vi "Main.vi"(10 "COMport name":refnum<visa-resource-name>, 11 "Module Admin":refnum<class "Delacor_lib_QMH_Module Admin.lvclass">) -> ()   [LabVIEW 2018, in "MB 01 switches Module.lvlib"]
doc: "This template is based off of the Queued Message Handler design pattern and the Queued Message Handler project template that ships with LabVIEW.\n\nThe main difference is that the queue is private to this module and communication between modules is performed via Broadcast and Request events.\n\nRequest events are wrapped in public API methods and are handled in the Event Handling Loop (EHL) of this VI. Any module can register for Broadcast events sent by this module. The EHL generates messages based on user interface actions.\n\nThe Message Handling Loop (MHL) processes messages generated by the EHL, or by other messages. The messages are string values, so new messages can be added easily to the Message Cases case structure in the MHL. Each message cluster can also provide an optional value for Message Data, which is a variant that can be converted to whatever message-specific data is required.\n_____\nBased on DQMH Project Template 6.0.0.91."
uses:
  MB 01 switches Module.lvlib
  <vilib>/Delacor/Delacor QMH/Libraries/Module Admin_class/Delacor_lib_QMH_Module Admin.lvclass
  Module Data--cluster.ctl
  <vilib>/NI/Modbus Library/API/Master/Modbus Master.lvclass
  <vilib>/Delacor/Delacor QMH/Libraries/Message Queue_class/Delacor_lib_QMH_Message Queue.lvclass/Delacor_lib_QMH_Message Queue.ctl
  Stop Argument--cluster.ctl
  <vilib>/Delacor/Delacor QMH/Libraries/Module Admin_class/Delacor_lib_QMH_Module Admin.lvclass/Delacor_lib_QMH_Module Admin.ctl
  MB01 Open Argument--cluster.ctl
  demux1-10_chan0 Argument--cluster.ctl
  MB01_eMICs Argument--cluster.ctl
  MB01 Close Argument--cluster.ctl
  JIG Reset Argument--cluster.ctl
  Read JIG trigger Argument--cluster.ctl
  Read JIG trigger (Reply Payload)--cluster.ctl
  SC enable OFF Argument--cluster.ctl
  demux1-10_chan1 Argument--cluster.ctl
  demux1-10_chan2 Argument--cluster.ctl
  demux1-10_chan3 Argument--cluster.ctl
  demux1-10_chan4 Argument--cluster.ctl
  demux1-10_chan5 Argument--cluster.ctl
  demux1-10_chan6 Argument--cluster.ctl
  demux1-10_chan7 Argument--cluster.ctl
  demux1-10_chan8 Argument--cluster.ctl
  demux1-10_chan9 Argument--cluster.ctl
  demux1-10_chan10 Argument--cluster.ctl
  SC enable ON Argument--cluster.ctl
  SET trigger value Argument--cluster.ctl
  <vilib>/Utility/miscctls.llb/LVPointTypeDef.ctl
  Instrument Drivers/LV_driver_MBrelay/type defs/FGV enum.ctl
  <vilib>/Delacor/Delacor QMH/Libraries/Message Queue_class/Delacor_lib_QMH_Enqueue Message (Single).vi
  <vilib>/Delacor/Delacor QMH/Libraries/Module Admin_class/Delacor_lib_QMH_Get External Launch.vi
  <vilib>/Utility/error.llb/Error Cluster From Error Code.vi
  <vilib>/ErrorRing/Error Ring.xnode
  <vilib>/Delacor/Delacor QMH/Libraries/Message Queue_class/Delacor_lib_QMH_Message Queue.lvclass
  Instrument Drivers/LV_driver_MBrelay/MB Relay.lvlib
panel:
  out "trigger value":bool
  out "error out":errorcluster
  out "Status":string
  in  "Simulate MHL Error":bool
  in  "Simulate EHL Error":bool
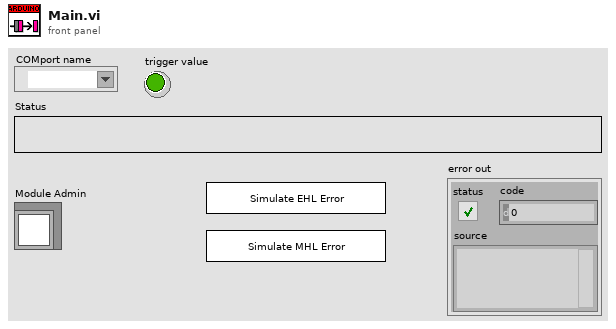
[diagram p1: front panel]
types:
  T1 = typedef "MB 01 switches Module.lvlib/Request Events--cluster.ctl" = cluster{"Stop Module":refnum<user-event>, "Show Panel":refnum<user-event>, "Hide Panel":refnum<user-event>, "Get Module Execution Status":refnum<user-event>, "Show Diagram":refnum<user-event>, "MB01 Open":refnum<user-event>, "demux1-10_chan0":refnum<user-event>, "MB01_eMICs":refnum<user-event>, "MB01 Close":refnum<user-event>, "JIG Reset":refnum<user-event>, "Read JIG trigger":refnum<user-event>, "SC enable OFF":refnum<user-event>, "demux1-10_chan1":refnum<user-event>, "demux1-10_chan2":refnum<user-event>, "demux1-10_chan3":refnum<user-event>, "demux1-10_chan4":refnum<user-event>, "demux1-10_chan5":refnum<user-event>, "demux1-10_chan6":refnum<user-event>, "demux1-10_chan7":refnum<user-event>, "demux1-10_chan8":refnum<user-event>, "demux1-10_chan9":refnum<user-event>, "demux1-10_chan10":refnum<user-event>, "SC enable ON":refnum<user-event>, "SET trigger value":refnum<user-event>}
  T2 = typedef "MB 01 switches Module.lvlib/Module Data--cluster.ctl" = cluster{"Status":string, "VISA resource name":refnum<visa-resource-name>, "Modbus Master out":refnum<class "Modbus Master.lvclass">}
  T3 = enum32{"invalid lock state", "Not Locked", "Locked (No Password)", "Password-protected"}
  T4 = typedef "MB 01 switches Module.lvlib/Stop Argument--cluster.ctl" = cluster{"Origin":string, "Exit via Stop Module Req?":bool, "Wait for Module to stop?":bool}
  T5 = typedef "MB 01 switches Module.lvlib/MB01 Open Argument--cluster.ctl" = cluster{"VISA resource name":refnum<visa-resource-name>}
  T6 = typedef "MB 01 switches Module.lvlib/demux1-10_chan0 Argument--cluster.ctl" = cluster{"demux1_10(x6)_encode":enum16{"demux1_10_channel0", "demux1_10_channel1", "demux1_10_channel2", "demux1_10_channel3", "demux1_10_channel4", "demux1_10_channel5", "demux1_10_channel6", "demux1_10_channel7", "demux1_10_channel8", "demux1_10_channel9", "demux1_10_channel10"}}
  T7 = typedef "MB 01 switches Module.lvlib/MB01_eMICs Argument--cluster.ctl" = cluster{"Array":bool[]}
  T8 = typedef "MB 01 switches Module.lvlib/MB01 Close Argument--cluster.ctl" = cluster{"Boolean":bool}
  T9 = typedef "MB 01 switches Module.lvlib/JIG Reset Argument--cluster.ctl" = cluster{"Boolean":bool}
  T10 = typedef "MB 01 switches Module.lvlib/Read JIG trigger Argument--cluster.ctl" = cluster{"Wait Notifier":refnum<notifier>, "wait for reply":bool}
  T11 = typedef "MB 01 switches Module.lvlib/SC enable OFF Argument--cluster.ctl" = cluster{"Boolean":bool}
  T12 = typedef "MB 01 switches Module.lvlib/demux1-10_chan1 Argument--cluster.ctl" = cluster{"Boolean":bool}
  T13 = typedef "MB 01 switches Module.lvlib/demux1-10_chan2 Argument--cluster.ctl" = cluster{"Boolean":bool}
  T14 = typedef "MB 01 switches Module.lvlib/demux1-10_chan3 Argument--cluster.ctl" = cluster{"Boolean":bool}
  T15 = typedef "MB 01 switches Module.lvlib/demux1-10_chan4 Argument--cluster.ctl" = cluster{"Boolean":bool}
  T16 = typedef "MB 01 switches Module.lvlib/demux1-10_chan5 Argument--cluster.ctl" = cluster{"Boolean":bool}
  T17 = typedef "MB 01 switches Module.lvlib/demux1-10_chan6 Argument--cluster.ctl" = cluster{"Boolean":bool}
  T18 = typedef "MB 01 switches Module.lvlib/demux1-10_chan7 Argument--cluster.ctl" = cluster{"Boolean":bool}
  T19 = typedef "MB 01 switches Module.lvlib/demux1-10_chan8 Argument--cluster.ctl" = cluster{"Boolean":bool}
  T20 = typedef "MB 01 switches Module.lvlib/demux1-10_chan9 Argument--cluster.ctl" = cluster{"Boolean":bool}
  T21 = typedef "MB 01 switches Module.lvlib/demux1-10_chan10 Argument--cluster.ctl" = cluster{"Boolean":bool}
  T22 = typedef "MB 01 switches Module.lvlib/SC enable ON Argument--cluster.ctl" = cluster{"Boolean":bool}
  T23 = typedef "MB 01 switches Module.lvlib/SET trigger value Argument--cluster.ctl" = cluster{"Boolean":bool}
  T24 = typedef "LVPointTypeDef.ctl" = cluster{"Horizontal":i16, "Vertical":i16}
  T25 = enum32{"Invalid", "Standard", "Closed", "Hidden", "Minimized", "Maximized"}
  T26 = typedef "MB Relay.lvlib/FGV enum.ctl" = enum16{"Write", "Init FGV", "Read", "All OFF", "All ON"}
  T27 = enum16{"demux1_10_channel0", "demux1_10_channel1", "demux1_10_channel2", "demux1_10_channel3", "demux1_10_channel4", "demux1_10_channel5", "demux1_10_channel6", "demux1_10_channel7", "demux1_10_channel8", "demux1_10_channel9", "demux1_10_channel10"}
  T28 = typedef "MB 01 switches Module.lvlib/Read JIG trigger (Reply Payload)--cluster.ctl" = cluster{"Trigger?":bool, "Read JIG trigger_error":errorcluster}
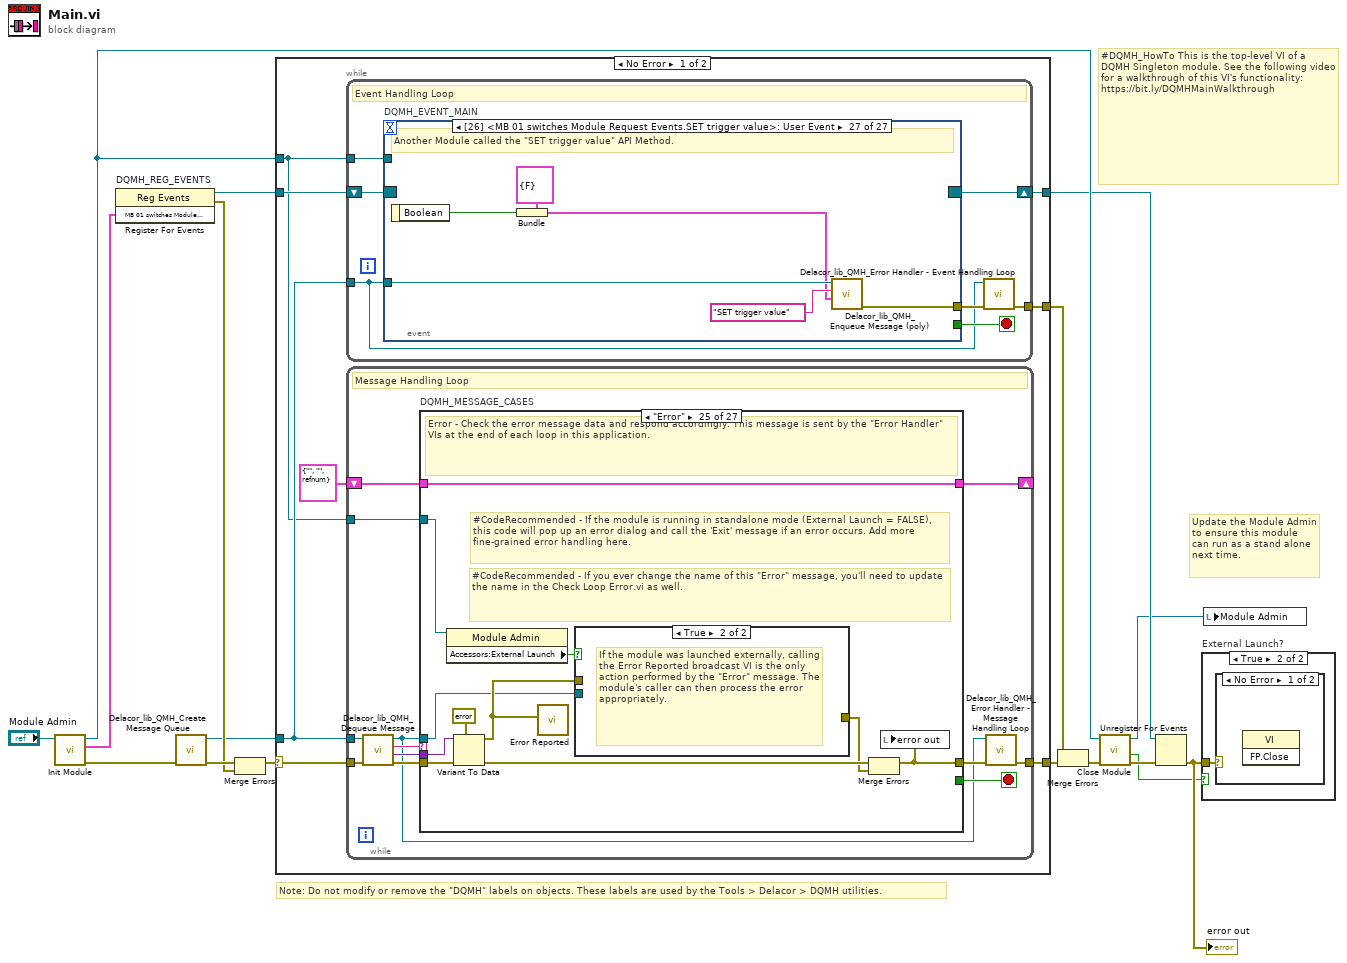
[diagram p0: block diagram]
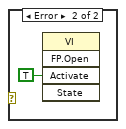
[diagram p3: hidden frame]
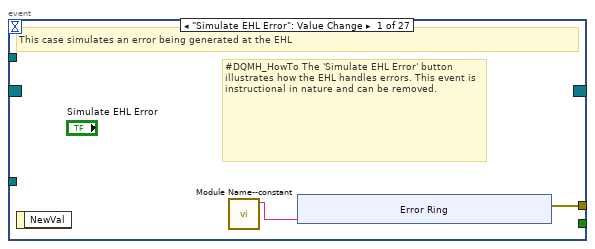
[diagram p4: hidden frame]
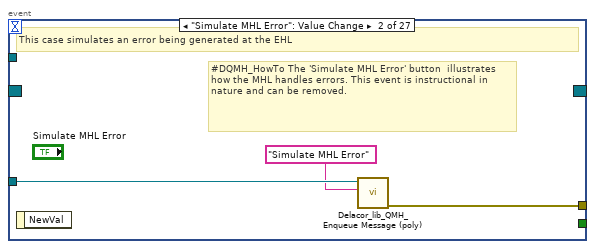
[diagram p5: hidden frame]
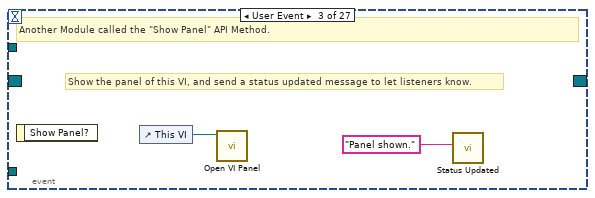
[diagram p6: hidden frame]
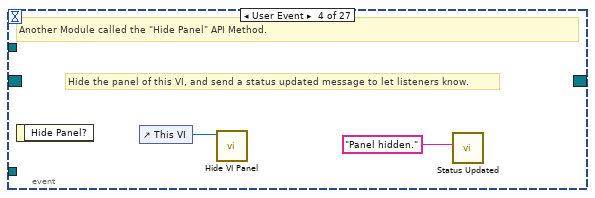
[diagram p7: hidden frame]
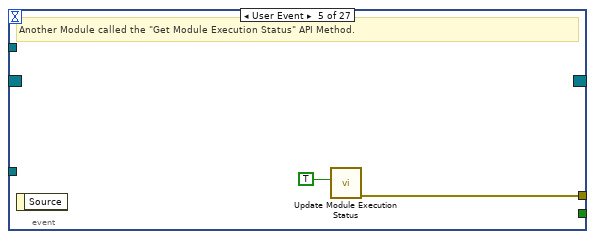
[diagram p8: hidden frame]
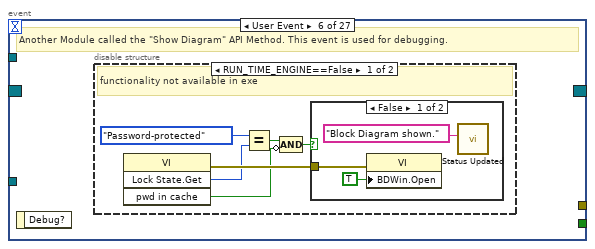
[diagram p9: hidden frame]
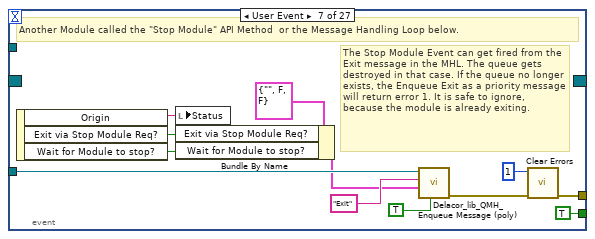
[diagram p12: hidden frame]
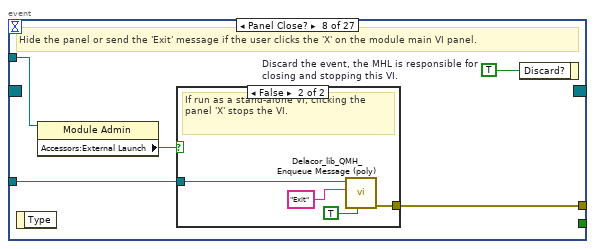
[diagram p13: hidden frame]
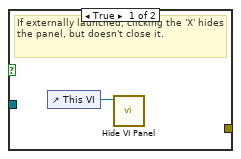
[diagram p14: hidden frame]
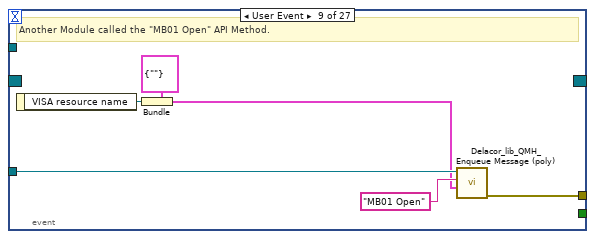
[diagram p15: hidden frame]
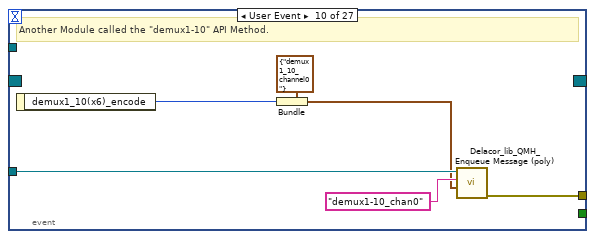
[diagram p16: hidden frame]
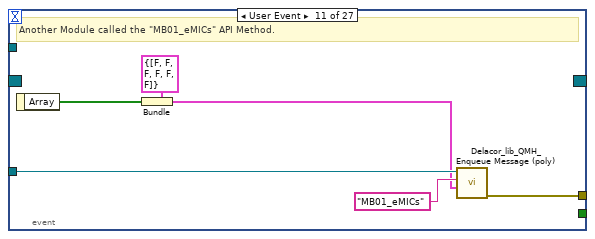
[diagram p17: hidden frame]
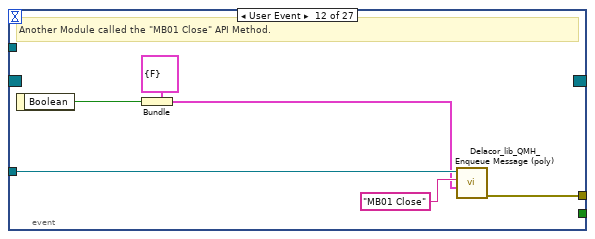
[diagram p18: hidden frame]
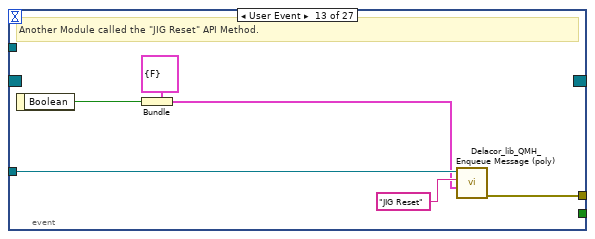
[diagram p19: hidden frame]
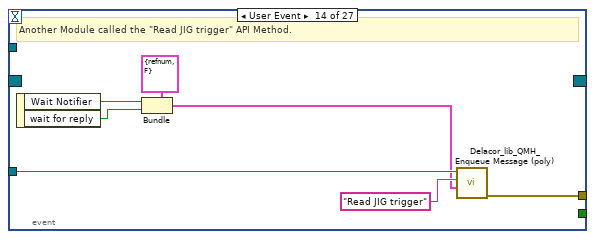
[diagram p20: hidden frame]
diagram:
  # "#DQMH_HowTo This is the top-level VI of a DQMH Singleton module. See the following video for a walkthrough of this VI's functionality: https://bit.ly/DQMHMainWalkthrough"
  # "Note: Do not modify or remove the \"DQMH\" labels on objects. These labels are used by the Tools > Delacor > DQMH utilities."
  # "Update the Module Admin to ensure this module can run as a stand alone next time."
  n1 = call "Init Module.vi"("Singleton Module Admin in"="Module Admin") -> ("error out"=w16:errorcluster, "MB 01 switches Module Request Events"=w5:T1, "Singleton Module Admin out"=w8:refnum<class "Delacor_lib_QMH_Module Admin.lvclass">)  [unwired: 8 in]
  n2 = register-events "DQMH_REG_EVENTS"(w5) -> (reference out=w6:refnum<event-registration>, error out=w9:errorcluster)  [unwired: 2 in]
  n3 = call <vilib>:"Delacor_lib_QMH_Create Message Queue.vi"("error in"=w16) -> ("error out"=w11:errorcluster, "Message Queue"=w4:refnum<class "Delacor_lib_QMH_Message Queue.lvclass">)  [unwired: 9 in]
  n4 = Merge Errors(w11, w9) -> (w10:errorcluster)
  n5 = case shown="No Error" w10 {
    selector: w10 -> [w23 w534]
    tunnel: [w25 w533] -> w17
    tunnel: [w22 w539] -> w7
    tunnel: w6 -> [w20 w539]
    tunnel: w4 -> [w19 w532]
    tunnel: [w24 _] -> w14
    tunnel: w8 -> [w18 w535]
    frame No Error {
      n6 = while {
        tunnel: w19 -> [w26]
        shift-right: [w29] -> w22
        shift-left: w20 -> [w30]
        tunnel: [w31] -> w24
        tunnel: w18 -> [w27]
        stop <- w28 stop-if-true
        # "Event Handling Loop"
        n7 = event "DQMH_EVENT_MAIN" shown="[26] <MB 01 switches Module Request Events.SET trigger value>: User Event" {
          selector: w30 -> [_ _ _ _ _ _ _ _ _ _ _ _ _ _ _ _ _ _ _ _ _ _ _ _ _ _ _]
          dyn-events: [_ _ _ _ _ _ _ _ _ _ _ _ _ _ _ _ _ _ _ _ _ _ _ _ _ _ _] -> w29
          timeout: _ -> [_ _ _ _ _ _ _ _ _ _ _ _ _ _ _ _ _ _ _ _ _ _ _ _ _ _ _]
          tunnel: [_ _ _ _ _ _ TRUE ("Discard?") _ _ _ _ _ _ _ _ _ _ _ _ _ _ _ _ _ _ _ _] -> w28
          tunnel: w26 -> [_ w43 _ _ _ _ w67 w74 w87 w93 w99 w105 w111 w118 w124 w130 w136 w142 w148 w154 w160 w166 w172 w178 w184 w190 w196]
          tunnel: [w34 w44 _ _ w50 _ w70 w76 w82 w88 w94 w100 w106 w112 w119 w125 w131 w137 w143 w149 w155 w161 w167 w173 w179 w185 w191] -> w32
          tunnel: w27 -> [_ _ _ _ _ _ _ w73 _ _ _ _ _ _ _ _ _ _ _ _ _ _ _ _ _ _ _]
          event "Simulate EHL Error": Value Change {
            # "#DQMH_HowTo The 'Simulate EHL Error' button  illustrates how the EHL handles errors. This event is instructional in nature and can be removed."
            # "This case simulates an error being generated at the EHL"
            n8 = event-data() -> ()  [unwired: 1 in, 1 out]
            n9 = call "Module Name--constant.vi"() -> ("Module Name"=w33:string)  [unwired: 11 in]
            n10 = xnode "Error Ring"("parameter 0"=w33) -> ("error out"=w34:errorcluster)
          }
          event "Simulate MHL Error": Value Change {
            # "#DQMH_HowTo The 'Simulate MHL Error' button  illustrates how the MHL handles errors. This event is instructional in nature and can be removed."
            # "This case simulates an error being generated at the EHL"
            n11 = event-data() -> ()  [unwired: 1 in, 1 out]
            n12 = call-poly <vilib>:"Delacor_lib_QMH_Enqueue Message (poly).vi"("Message"="Simulate MHL Error", "Message Queue in"=w43) -> ("error out"=w44:errorcluster)  [unwired: 8 in, 1 out]
          }
          event User Event {
            # "Show the panel of this VI, and send a status updated message to let listeners know."
            # "Another Module called the \"Show Panel\" API Method."
            n13 = event-data() -> ()  [unwired: 1 in, 1 out]
            n14 = control-ref of="This VI"() -> (w46:refnum<vi>)
            n15 = call "Open VI Panel.vi"("VI"=w46) -> ()  [unwired: 10 in, 1 out]
            n16 = call "Status Updated.vi"("Status"="Panel shown." ("format string")) -> ()  [unwired: 10 in, 1 out]
          }
          event User Event {
            # "Hide the panel of this VI, and send a status updated message to let listeners know."
            # "Another Module called the \"Hide Panel\" API Method."
            n17 = event-data() -> ()  [unwired: 1 in, 1 out]
            n18 = control-ref of="This VI"() -> (w48:refnum<vi>)
            n19 = call "Hide VI Panel.vi"("VI"=w48) -> ()  [unwired: 10 in, 1 out]
            n20 = call "Status Updated.vi"("Status"="Panel hidden." ("format string")) -> ()  [unwired: 10 in, 1 out]
          }
          event User Event {
            # "Another Module called the \"Get Module Execution Status\" API Method."
            n21 = event-data() -> ()  [unwired: 1 in, 1 out]
            n22 = call "Update Module Execution Status.vi"("Running?"=TRUE) -> ("error out"=w50:errorcluster)  [unwired: 10 in]
          }
          event User Event {
            # "Another Module called the \"Show Diagram\" API Method. This event is used for debugging."
            n23 = event-data() -> ()  [unwired: 1 in, 1 out]
            n24 = disable-structure shown="RUN_TIME_ENGINE==False" {
              frame condition #0 (active) {
                # "functionality not available in exe"
                n25 = invoke class="VI" method="Lock State.Get"() -> (error out=w56:errorcluster, "Get Lock State"=w55:T3, "pwd in cache"=w52:bool)  [unwired: 4 in, 1 out]
                n26 = Equal?(x=T3."Password-protected", y=w55) -> (x = y?=w53:bool)
                n27 = Compound Arithmetic op=AND(w53, invert w52) -> (w51:bool)
                n28 = case shown="False" w51 {
                  tunnel: w56 -> [w59 _]
                  frame False {
                    n29 = property class="VI"(error in=w59, "BDWin.Open"=TRUE ("Block Diagram Window:Open")) -> ()  [unwired: 1 in, 2 out]
                    n30 = call "Status Updated.vi"("Status"="Block Diagram shown." ("format string")) -> ()  [unwired: 10 in, 1 out]
                  }
                  frame True {
                    # "Password-protected VI, and the password is not in the cache. Do not show the diagram."
                  }
                }
              }
              frame condition #1 {
              }
            }
          }
          event User Event {
            # "The Stop Module Event can get fired from the Exit message in the MHL. The queue gets destroyed in that case. If the queue no longer exists, the Enqueue Exit as a priority message will return error 1. It is safe to ignore, because the module is already exiting."
            # "Another Module called the \"Stop Module\" API Method  or the Message Handling Loop below."
            n31 = event-data() -> ("Origin"=w66:string, "Exit via Stop Module Req?"=w62:bool, "Wait for Module to stop?"=w61:bool)  [unwired: 1 in]
            n32 = local write "Status"(w66) -> ()
            n33 = Bundle By Name(cluster=T4 {"Origin"="", "Exit via Stop Module Req?"=FALSE, "Wait for Module to stop?"=FALSE} ("Stop Argument"), "Exit via Stop Module Req?"=w62, "Wait for Module to stop?"=w61) -> (w60:T4)
            n34 = call-poly <vilib>:"Delacor_lib_QMH_Enqueue Message (poly).vi"("Priority Message? (F)"=TRUE, "Message Data"=w60, "Message"="Exit", "Message Queue in"=w67) -> ("error out"=w71:errorcluster)  [unwired: 6 in, 1 out]
            n35 = call <vilib>:"Clear Errors.vi"("error in (no error)"=w71, "specific error code to clear (0: all)"=1) -> ("error out"=w70:errorcluster)  [unwired: 4 in, 1 out]
          }
          event Panel Close? {
            w75 = TRUE  # Discard the event, the MHL is responsible for closing and stopping this VI.
            # "Hide the panel or send the 'Exit' message if the user clicks the 'X' on the module main VI panel."
            n36 = event-data() -> ()  [unwired: 1 in, 1 out]
            n37 = property class="Module Admin"(reference=w73) -> ("Accessors:External Launch"=w72:bool)  [unwired: 1 in, 2 out]
            n38 = case shown="False" w72 {
              tunnel: w74 -> [_ w80]
              tunnel: [_ w81] -> w76
              frame True {
                # "If externally launched, clicking the 'X' hides the panel, but doesn't close it."
                n39 = control-ref of="This VI"() -> (w77:refnum<vi>)
                n40 = call "Hide VI Panel.vi"("VI"=w77) -> ()  [unwired: 10 in, 1 out]
              }
              frame False {
                # "If run as a stand-alone VI, clicking the panel 'X' stops the VI."
                n41 = call-poly <vilib>:"Delacor_lib_QMH_Enqueue Message (poly).vi"("Priority Message? (F)"=TRUE, "Message"="Exit", "Message Queue in"=w80) -> ("error out"=w81:errorcluster)  [unwired: 7 in, 1 out]
              }
            }
            n42 = event-data("Discard?"=w75) -> ()  [unwired: 1 in, 1 out]
          }
          event User Event {
            # "Another Module called the \"MB01 Open\" API Method."
            n43 = event-data() -> ("VISA resource name"=w83:refnum<visa-resource-name>)  [unwired: 1 in]
            n44 = Bundle(cluster=T5 {"VISA resource name"=""} ("MB01 Open Argument"), "VISA resource name"=w83) -> (w84:T5)
            n45 = call-poly <vilib>:"Delacor_lib_QMH_Enqueue Message (poly).vi"("Message Data"=w84, "Message"="MB01 Open", "Message Queue in"=w87) -> ("error out"=w82:errorcluster)  [unwired: 7 in, 1 out]
          }
          event User Event {
            # "Another Module called the \"demux1-10\" API Method."
            n46 = event-data() -> ("demux1_10(x6)_encode"=w89:T27)  [unwired: 1 in]
            n47 = Bundle(cluster=T6 {"demux1_10(x6)_encode"=enum."demux1_10_channel0"} ("demux1-10 Argument"), "demux1_10(x6)_encode"=w89) -> (w90:T6)
            n48 = call-poly <vilib>:"Delacor_lib_QMH_Enqueue Message (poly).vi"("Message Data"=w90, "Message"="demux1-10_chan0", "Message Queue in"=w93) -> ("error out"=w88:errorcluster)  [unwired: 7 in, 1 out]
          }
          event User Event {
            # "Another Module called the \"MB01_eMICs\" API Method."
            n49 = event-data() -> ("Array"=w95:bool[])  [unwired: 1 in]
            n50 = Bundle(cluster=T7 {"Array"=[FALSE, FALSE, FALSE, FALSE, FALSE, FALSE]} ("MB01_eMICs Argument"), "Array"=w95) -> (w96:T7)
            n51 = call-poly <vilib>:"Delacor_lib_QMH_Enqueue Message (poly).vi"("Message Data"=w96, "Message"="MB01_eMICs", "Message Queue in"=w99) -> ("error out"=w94:errorcluster)  [unwired: 7 in, 1 out]
          }
          event User Event {
            # "Another Module called the \"MB01 Close\" API Method."
            n52 = event-data() -> ("Boolean"=w101:bool)  [unwired: 1 in]
            n53 = Bundle(cluster=T8 {"Boolean"=FALSE} ("MB01 Close Argument"), "Boolean"=w101) -> (w102:T8)
            n54 = call-poly <vilib>:"Delacor_lib_QMH_Enqueue Message (poly).vi"("Message Data"=w102, "Message"="MB01 Close", "Message Queue in"=w105) -> ("error out"=w100:errorcluster)  [unwired: 7 in, 1 out]
          }
          event User Event {
            # "Another Module called the \"JIG Reset\" API Method."
            n55 = event-data() -> ("Boolean"=w107:bool)  [unwired: 1 in]
            n56 = Bundle(cluster=T9 {"Boolean"=FALSE} ("JIG Reset Argument"), "Boolean"=w107) -> (w108:T9)
            n57 = call-poly <vilib>:"Delacor_lib_QMH_Enqueue Message (poly).vi"("Message Data"=w108, "Message"="JIG Reset", "Message Queue in"=w111) -> ("error out"=w106:errorcluster)  [unwired: 7 in, 1 out]
          }
          event User Event {
            # "Another Module called the \"Read JIG trigger\" API Method."
            n58 = event-data() -> ("Wait Notifier"=w114:refnum<notifier>, "wait for reply"=w113:bool)  [unwired: 1 in]
            n59 = Bundle(cluster=T10 {"Wait Notifier"=refnum, "wait for reply"=FALSE} ("Read JIG trigger Argument"), "Wait Notifier"=w114, "wait for reply"=w113) -> (w115:T10)
            n60 = call-poly <vilib>:"Delacor_lib_QMH_Enqueue Message (poly).vi"("Message Data"=w115, "Message"="Read JIG trigger", "Message Queue in"=w118) -> ("error out"=w112:errorcluster)  [unwired: 7 in, 1 out]
          }
          event User Event {
            # "Another Module called the \"SC enable OFF\" API Method."
            n61 = event-data() -> ("Boolean"=w120:bool)  [unwired: 1 in]
            n62 = Bundle(cluster=T11 {"Boolean"=FALSE} ("SC enable OFF Argument"), "Boolean"=w120) -> (w121:T11)
            n63 = call-poly <vilib>:"Delacor_lib_QMH_Enqueue Message (poly).vi"("Message Data"=w121, "Message"="SC enable OFF", "Message Queue in"=w124) -> ("error out"=w119:errorcluster)  [unwired: 7 in, 1 out]
          }
          event User Event {
            # "Another Module called the \"demux1-10_chan1\" API Method."
            n64 = event-data() -> ("Boolean"=w126:bool)  [unwired: 1 in]
            n65 = Bundle(cluster=T12 {"Boolean"=FALSE} ("demux1-10_chan1 Argument"), "Boolean"=w126) -> (w127:T12)
            n66 = call-poly <vilib>:"Delacor_lib_QMH_Enqueue Message (poly).vi"("Message Data"=w127, "Message"="demux1-10_chan1", "Message Queue in"=w130) -> ("error out"=w125:errorcluster)  [unwired: 7 in, 1 out]
          }
          event User Event {
            # "Another Module called the \"demux1-10_chan2\" API Method."
            n67 = event-data() -> ("Boolean"=w132:bool)  [unwired: 1 in]
            n68 = Bundle(cluster=T13 {"Boolean"=FALSE} ("demux1-10_chan2 Argument"), "Boolean"=w132) -> (w133:T13)
            n69 = call-poly <vilib>:"Delacor_lib_QMH_Enqueue Message (poly).vi"("Message Data"=w133, "Message"="demux1-10_chan2", "Message Queue in"=w136) -> ("error out"=w131:errorcluster)  [unwired: 7 in, 1 out]
          }
          event User Event {
            # "Another Module called the \"demux1-10_chan3\" API Method."
            n70 = event-data() -> ("Boolean"=w138:bool)  [unwired: 1 in]
            n71 = Bundle(cluster=T14 {"Boolean"=FALSE} ("demux1-10_chan3 Argument"), "Boolean"=w138) -> (w139:T14)
            n72 = call-poly <vilib>:"Delacor_lib_QMH_Enqueue Message (poly).vi"("Message Data"=w139, "Message"="demux1-10_chan3", "Message Queue in"=w142) -> ("error out"=w137:errorcluster)  [unwired: 7 in, 1 out]
          }
          event User Event {
            # "Another Module called the \"demux1-10_chan4\" API Method."
            n73 = event-data() -> ("Boolean"=w144:bool)  [unwired: 1 in]
            n74 = Bundle(cluster=T15 {"Boolean"=FALSE} ("demux1-10_chan4 Argument"), "Boolean"=w144) -> (w145:T15)
            n75 = call-poly <vilib>:"Delacor_lib_QMH_Enqueue Message (poly).vi"("Message Data"=w145, "Message"="demux1-10_chan4", "Message Queue in"=w148) -> ("error out"=w143:errorcluster)  [unwired: 7 in, 1 out]
          }
          event User Event {
            # "Another Module called the \"demux1-10_chan5\" API Method."
            n76 = event-data() -> ("Boolean"=w150:bool)  [unwired: 1 in]
            n77 = Bundle(cluster=T16 {"Boolean"=FALSE} ("demux1-10_chan5 Argument"), "Boolean"=w150) -> (w151:T16)
            n78 = call-poly <vilib>:"Delacor_lib_QMH_Enqueue Message (poly).vi"("Message Data"=w151, "Message"="demux1-10_chan5", "Message Queue in"=w154) -> ("error out"=w149:errorcluster)  [unwired: 7 in, 1 out]
          }
          event User Event {
            # "Another Module called the \"demux1-10_chan6\" API Method."
            n79 = event-data() -> ("Boolean"=w156:bool)  [unwired: 1 in]
            n80 = Bundle(cluster=T17 {"Boolean"=FALSE} ("demux1-10_chan6 Argument"), "Boolean"=w156) -> (w157:T17)
            n81 = call-poly <vilib>:"Delacor_lib_QMH_Enqueue Message (poly).vi"("Message Data"=w157, "Message"="demux1-10_chan6", "Message Queue in"=w160) -> ("error out"=w155:errorcluster)  [unwired: 7 in, 1 out]
          }
          event User Event {
            # "Another Module called the \"demux1-10_chan7\" API Method."
            n82 = event-data() -> ("Boolean"=w162:bool)  [unwired: 1 in]
            n83 = Bundle(cluster=T18 {"Boolean"=FALSE} ("demux1-10_chan7 Argument"), "Boolean"=w162) -> (w163:T18)
            n84 = call-poly <vilib>:"Delacor_lib_QMH_Enqueue Message (poly).vi"("Message Data"=w163, "Message"="demux1-10_chan7", "Message Queue in"=w166) -> ("error out"=w161:errorcluster)  [unwired: 7 in, 1 out]
          }
          event User Event {
            # "Another Module called the \"demux1-10_chan8\" API Method."
            n85 = event-data() -> ("Boolean"=w168:bool)  [unwired: 1 in]
            n86 = Bundle(cluster=T19 {"Boolean"=FALSE} ("demux1-10_chan8 Argument"), "Boolean"=w168) -> (w169:T19)
            n87 = call-poly <vilib>:"Delacor_lib_QMH_Enqueue Message (poly).vi"("Message Data"=w169, "Message"="demux1-10_chan8", "Message Queue in"=w172) -> ("error out"=w167:errorcluster)  [unwired: 7 in, 1 out]
          }
          event User Event {
            # "Another Module called the \"demux1-10_chan9\" API Method."
            n88 = event-data() -> ("Boolean"=w174:bool)  [unwired: 1 in]
            n89 = Bundle(cluster=T20 {"Boolean"=FALSE} ("demux1-10_chan9 Argument"), "Boolean"=w174) -> (w175:T20)
            n90 = call-poly <vilib>:"Delacor_lib_QMH_Enqueue Message (poly).vi"("Message Data"=w175, "Message"="demux1-10_chan9", "Message Queue in"=w178) -> ("error out"=w173:errorcluster)  [unwired: 7 in, 1 out]
          }
          event User Event {
            # "Another Module called the \"demux1-10_chan10\" API Method."
            n91 = event-data() -> ("Boolean"=w180:bool)  [unwired: 1 in]
            n92 = Bundle(cluster=T21 {"Boolean"=FALSE} ("demux1-10_chan10 Argument"), "Boolean"=w180) -> (w181:T21)
            n93 = call-poly <vilib>:"Delacor_lib_QMH_Enqueue Message (poly).vi"("Message Data"=w181, "Message"="demux1-10_chan10", "Message Queue in"=w184) -> ("error out"=w179:errorcluster)  [unwired: 7 in, 1 out]
          }
          event User Event {
            # "Another Module called the \"SC enable ON\" API Method."
            n94 = event-data() -> ("Boolean"=w186:bool)  [unwired: 1 in]
            n95 = Bundle(cluster=T22 {"Boolean"=FALSE} ("SC enable ON Argument"), "Boolean"=w186) -> (w187:T22)
            n96 = call-poly <vilib>:"Delacor_lib_QMH_Enqueue Message (poly).vi"("Message Data"=w187, "Message"="SC enable ON", "Message Queue in"=w190) -> ("error out"=w185:errorcluster)  [unwired: 7 in, 1 out]
          }
          event User Event {
            # "Another Module called the \"SET trigger value\" API Method."
            n97 = event-data() -> ("Boolean"=w192:bool)  [unwired: 1 in]
            n98 = Bundle(cluster=T23 {"Boolean"=FALSE} ("SET trigger value Argument"), "Boolean"=w192) -> (w193:T23)
            n99 = call-poly <vilib>:"Delacor_lib_QMH_Enqueue Message (poly).vi"("Message Data"=w193, "Message"="SET trigger value", "Message Queue in"=w196) -> ("error out"=w191:errorcluster)  [unwired: 7 in, 1 out]
          }
        }
        n100 = call-dynamic "Delacor_lib_QMH_Error Handler - Event Handling Loop.vi"("error in"=w32, "Message Queue in"=w26) -> ("dup error in"=w31:errorcluster)  [unwired: 8 in, 1 out]
      }
      n101 = while {
        tunnel: w19 -> [w199]
        shift-right: [w203] -> _
        shift-left: T2 {"Status"="", "VISA resource name"="", "Modbus Master out"=refnum} ("Data Cluster") -> [w204]
        tunnel: w23 -> [w207]
        tunnel: [w205] -> w25
        tunnel: w18 -> [w197]
        stop <- w202 stop-if-true
        # "Message Handling Loop"
        n102 = call-dynamic "Delacor_lib_QMH_Dequeue Message.vi"("error in"=w207, "Message Queue in"=w199) -> ("error out"=w206:errorcluster, "Message Data"=w200:variant, "Message"=w201:string, "Message Queue out"=w198:refnum<class "Delacor_lib_QMH_Message Queue.lvclass">)  [unwired: 6 in]
        n103 = case "DQMH_MESSAGE_CASES" shown="\"Error\"" w201 {
          selector: w201 -> [_ _ _ _ _ _ _ _ _ _ _ _ _ _ _ _ _ _ _ _ _ _ _ _ _ _ w519]
          tunnel: w198 -> [_ _ _ _ _ _ _ _ _ _ _ _ _ _ _ _ _ _ _ _ _ _ _ _ w482 w505 _]
          tunnel: w206 -> [w214 w230 w242 w254 w267 w278 w289 w300 w311 w322 w333 w344 w355 w366 w377 w389 w401 w412 w437 w451 w462 w465 w467 w472 w489 w511 w521]
          tunnel: [w213 w230 w236 w248 w261 w273 w284 w295 w306 w317 w328 w339 w350 w361 w372 w382 w396 w407 w428 w446 w460 w464 w467 w471 w485 w508 w522] -> w208
          tunnel: w204 -> [w210 w229 w235 w251 w264 w274 w285 w296 w307 w318 w329 w340 w351 w362 w373 w385 w397 w409 w427 w447 w461 w463 w466 w469 w484 w497 w520]
          tunnel: [w218 w229 w238 w251 w264 w274 w285 w296 w307 w318 w329 w340 w351 w362 w373 w385 w397 w409 w427 w447 w461 w463 w466 w469 w484 w497 w520] -> w203
          tunnel: [_ _ _ _ _ _ _ _ _ _ _ _ _ _ _ _ _ _ _ _ _ _ _ _ _ w504 _] -> w202
          tunnel: w200 -> [_ _ w241 w253 w266 w276 w287 w298 w309 w320 w331 w342 w353 w364 w375 w388 w399 w411 w435 w449 w459 _ _ _ w483 w503 _]
          tunnel: w197 -> [w219 _ _ _ _ _ _ _ _ _ _ _ _ _ _ _ _ _ _ _ _ _ _ _ w481 w498 _]
          frame "Initialize" {
            w216 = "Initial Message" ("Initial Message")
            # "Initialize - Any operation that needs to be done before the module can receive messages. Synchronize Caller Events.vi will inform Start Module.vi that the module has launched and is ready to receive messages. Module Did Init.vi will broadcast that the module initialized."
            n104 = call "Synchronize Caller Events.vi"("error in (no error)"=w214, "Singleton Module Admin in"=w219) -> ("error out"=w209:errorcluster, "Singleton Module Admin out"=w217:refnum<class "Delacor_lib_QMH_Module Admin.lvclass">)  [unwired: 8 in]
            n105 = property class="Module Admin"(reference=w217) -> ("Accessors:External Launch"=w223:bool)  [unwired: 1 in, 2 out]
            n106 = Bundle By Name(cluster=w210, "VISA resource name"="COMport name") -> (w211:T2)
            n107 = Select(t=T25."Hidden" ("State"), s=w223, f=T25."Standard" ("State")) -> (s? t:f=w220:T25)
            n108 = call "Module Name--constant.vi"() -> ("Module Name"=w226:string)  [unwired: 11 in]
            n109 = property class="VI"("Front Panel.Title"=w226) -> (reference out=w225:refnum<vi>, error out=w228:errorcluster)  [unwired: 2 in]
            n110 = property on="Pane" class="Pane"("Origin"=T24 {"Horizontal"=0, "Vertical"=0}) -> ()  [unwired: 2 in, 2 out]
            n111 = invoke class="VI" method="FP.Open"(reference=w225, error in=w228, "State"=w220) -> (reference out=w224:refnum<vi>, error out=w227:errorcluster)  [unwired: 2 in, 3 out]
            n112 = Merge Errors(w209) -> (w213:errorcluster)
            n113 = invoke class="VI" method="FP.Center"(reference=w224, error in=w227) -> ()  [unwired: 1 in, 3 out]
            n114 = Bundle By Name(cluster=w211, "Status"=w216) -> (w218:T2)
            "Status" <- w216
          }
          frame "---Module Specific---" {
            # "Separator -- The following cases handle messages specific to this Module."
          }
          frame "MB01 Open" {
            # "Open Mobus on MB01"
            n115 = Variant To Data(error in=w242, type=T5 {"VISA resource name"=""} ("MB01 Open Argument"), Variant=w241) -> (error out=w237:errorcluster)  [unwired: 1 out]
            n116 = disable-structure shown="Default" {
              disable-tunnel: [w246 _] -> w239
              disable-tunnel: [w245 _] -> w232
              disable-tunnel: w235 -> [w244 _]
              frame condition #0 (active) {
                n117 = Unbundle By Name(w244) -> ("VISA resource name"=w243:refnum<visa-resource-name>)
                n118 = call "inst.Open.vi"("unit ID in"=u8 1, "VISA resource name"=w243) -> ("error out"=w245:errorcluster, "Modbus Master out"=w246:refnum<class "Modbus Master.lvclass">)  [unwired: 8 in]
              }
              frame condition #1 {
              }
            }
            n119 = Bundle By Name(cluster=w235, "Modbus Master out"=w239) -> (w238:T2)
            n120 = call "Module Name--constant.vi"() -> ("Module Name"=w234:string)  [unwired: 11 in]
            n121 = call "Module Did Init.vi"("error in (no error)"=w232, "Initialized?"=TRUE, "Origin"=w234) -> ("error out"=w231:errorcluster)  [unwired: 8 in]
            n122 = Merge Errors(w237, w231) -> (w236:errorcluster)
          }
          frame "MB01 Close" {
            # "Close COM port to MB01"
            n123 = Variant To Data(error in=w254, type=T8 {"Boolean"=FALSE} ("MB01 Close Argument"), Variant=w253) -> (error out=w249:errorcluster)  [unwired: 1 out]
            n124 = disable-structure shown="Default" {
              disable-tunnel: w251 -> [w260 _]
              disable-tunnel: [w259 _] -> w250
              frame condition #0 (active) {
                n125 = Unbundle By Name(w260) -> ("Modbus Master out"=w257:refnum<class "Modbus Master.lvclass">)
                n126 = call "FGV_HoldingRegs.vi"("FGV_enum"=FGV_enum."All OFF", "Modbus master in"=w257) -> ("error out"=w255:errorcluster, "Modbus master out"=w256:refnum<class "Modbus Master.lvclass">)  [unwired: 7 in, 1 out]
                n127 = call "inst.Close (SubVI).vi"("error in (no error)"=w255, "Modbus Master in"=w256) -> ("error out"=w259:errorcluster)  [unwired: 9 in]
              }
              frame condition #1 {
              }
            }
            n128 = Merge Errors(w249, w250) -> (w248:errorcluster)
          }
          frame "demux1-10_chan0" {
            # "Control demux 1-10 ( AC switches)"
            n129 = Variant To Data(error in=w267, type=T6 {"demux1_10(x6)_encode"=enum."demux1_10_channel0"} ("demux1-10 Argument"), Variant=w266) -> (error out=w262:errorcluster)  [unwired: 1 out]
            n130 = disable-structure shown="Default" {
              disable-tunnel: w264 -> [w271 _]
              disable-tunnel: [w269 _] -> w263
              frame condition #0 (active) {
                n131 = Unbundle By Name(w271) -> ("Modbus Master out"=w270:refnum<class "Modbus Master.lvclass">)
                n132 = call "inst.demux1.10(x6).vi"("demux1_10(x6)_encode"=T27."demux1_10_channel0", "Modbus Master in"=w270) -> ("error out"=w269:errorcluster)  [unwired: 8 in, 1 out]
              }
              frame condition #1 {
              }
            }
            n133 = Merge Errors(w262, w263) -> (w261:errorcluster)
          }
          frame "demux1-10_chan1" {
            n134 = Variant To Data(error in=w278, type=T12 {"Boolean"=FALSE} ("demux1-10_chan1 Argument"), Variant=w276) -> (error out=w277:errorcluster)  [unwired: 1 out]
            n135 = disable-structure shown="Default" {
              disable-tunnel: w274 -> [w282 _]
              disable-tunnel: [w279 _] -> w272
              frame condition #0 (active) {
                n136 = Unbundle By Name(w282) -> ("Modbus Master out"=w281:refnum<class "Modbus Master.lvclass">)
                n137 = call "inst.demux1.10(x6).vi"("demux1_10(x6)_encode"=T27."demux1_10_channel1", "Modbus Master in"=w281) -> ("error out"=w279:errorcluster)  [unwired: 8 in, 1 out]
              }
              frame condition #1 {
              }
            }
            n138 = Merge Errors(w277, w272) -> (w273:errorcluster)
          }
          frame "demux1-10_chan2" {
            n139 = Variant To Data(error in=w289, type=T13 {"Boolean"=FALSE} ("demux1-10_chan2 Argument"), Variant=w287) -> (error out=w288:errorcluster)  [unwired: 1 out]
            n140 = disable-structure shown="Default" {
              disable-tunnel: w285 -> [w293 _]
              disable-tunnel: [w290 _] -> w283
              frame condition #0 (active) {
                n141 = Unbundle By Name(w293) -> ("Modbus Master out"=w292:refnum<class "Modbus Master.lvclass">)
                n142 = call "inst.demux1.10(x6).vi"("demux1_10(x6)_encode"=T27."demux1_10_channel2", "Modbus Master in"=w292) -> ("error out"=w290:errorcluster)  [unwired: 8 in, 1 out]
              }
              frame condition #1 {
              }
            }
            n143 = Merge Errors(w288, w283) -> (w284:errorcluster)
          }
          frame "demux1-10_chan3" {
            n144 = Variant To Data(error in=w300, type=T14 {"Boolean"=FALSE} ("demux1-10_chan3 Argument"), Variant=w298) -> (error out=w299:errorcluster)  [unwired: 1 out]
            n145 = disable-structure shown="Default" {
              disable-tunnel: w296 -> [w304 _]
              disable-tunnel: [w301 _] -> w294
              frame condition #0 (active) {
                n146 = Unbundle By Name(w304) -> ("Modbus Master out"=w303:refnum<class "Modbus Master.lvclass">)
                n147 = call "inst.demux1.10(x6).vi"("demux1_10(x6)_encode"=T27."demux1_10_channel3", "Modbus Master in"=w303) -> ("error out"=w301:errorcluster)  [unwired: 8 in, 1 out]
              }
              frame condition #1 {
              }
            }
            n148 = Merge Errors(w299, w294) -> (w295:errorcluster)
          }
          frame "demux1-10_chan4" {
            n149 = Variant To Data(error in=w311, type=T15 {"Boolean"=FALSE} ("demux1-10_chan4 Argument"), Variant=w309) -> (error out=w310:errorcluster)  [unwired: 1 out]
            n150 = disable-structure shown="Default" {
              disable-tunnel: w307 -> [w315 _]
              disable-tunnel: [w312 _] -> w305
              frame condition #0 (active) {
                n151 = Unbundle By Name(w315) -> ("Modbus Master out"=w314:refnum<class "Modbus Master.lvclass">)
                n152 = call "inst.demux1.10(x6).vi"("demux1_10(x6)_encode"=T27."demux1_10_channel4", "Modbus Master in"=w314) -> ("error out"=w312:errorcluster)  [unwired: 8 in, 1 out]
              }
              frame condition #1 {
              }
            }
            n153 = Merge Errors(w310, w305) -> (w306:errorcluster)
          }
          frame "demux1-10_chan5" {
            n154 = Variant To Data(error in=w322, type=T16 {"Boolean"=FALSE} ("demux1-10_chan5 Argument"), Variant=w320) -> (error out=w321:errorcluster)  [unwired: 1 out]
            n155 = disable-structure shown="Default" {
              disable-tunnel: w318 -> [w326 _]
              disable-tunnel: [w323 _] -> w316
              frame condition #0 (active) {
                n156 = Unbundle By Name(w326) -> ("Modbus Master out"=w325:refnum<class "Modbus Master.lvclass">)
                n157 = call "inst.demux1.10(x6).vi"("demux1_10(x6)_encode"=T27."demux1_10_channel5", "Modbus Master in"=w325) -> ("error out"=w323:errorcluster)  [unwired: 8 in, 1 out]
              }
              frame condition #1 {
              }
            }
            n158 = Merge Errors(w321, w316) -> (w317:errorcluster)
          }
          frame "demux1-10_chan6" {
            n159 = Variant To Data(error in=w333, type=T17 {"Boolean"=FALSE} ("demux1-10_chan6 Argument"), Variant=w331) -> (error out=w332:errorcluster)  [unwired: 1 out]
            n160 = disable-structure shown="Default" {
              disable-tunnel: w329 -> [w337 _]
              disable-tunnel: [w334 _] -> w327
              frame condition #0 (active) {
                n161 = Unbundle By Name(w337) -> ("Modbus Master out"=w336:refnum<class "Modbus Master.lvclass">)
                n162 = call "inst.demux1.10(x6).vi"("demux1_10(x6)_encode"=T27."demux1_10_channel6", "Modbus Master in"=w336) -> ("error out"=w334:errorcluster)  [unwired: 8 in, 1 out]
              }
              frame condition #1 {
              }
            }
            n163 = Merge Errors(w332, w327) -> (w328:errorcluster)
          }
          frame "demux1-10_chan7" {
            n164 = Variant To Data(error in=w344, type=T18 {"Boolean"=FALSE} ("demux1-10_chan7 Argument"), Variant=w342) -> (error out=w343:errorcluster)  [unwired: 1 out]
            n165 = disable-structure shown="Default" {
              disable-tunnel: w340 -> [w348 _]
              disable-tunnel: [w345 _] -> w338
              frame condition #0 (active) {
                n166 = Unbundle By Name(w348) -> ("Modbus Master out"=w347:refnum<class "Modbus Master.lvclass">)
                n167 = call "inst.demux1.10(x6).vi"("demux1_10(x6)_encode"=T27."demux1_10_channel7", "Modbus Master in"=w347) -> ("error out"=w345:errorcluster)  [unwired: 8 in, 1 out]
              }
              frame condition #1 {
              }
            }
            n168 = Merge Errors(w343, w338) -> (w339:errorcluster)
          }
          frame "demux1-10_chan8" {
            n169 = Variant To Data(error in=w355, type=T19 {"Boolean"=FALSE} ("demux1-10_chan8 Argument"), Variant=w353) -> (error out=w354:errorcluster)  [unwired: 1 out]
            n170 = disable-structure shown="Default" {
              disable-tunnel: w351 -> [w359 _]
              disable-tunnel: [w356 _] -> w349
              frame condition #0 (active) {
                n171 = Unbundle By Name(w359) -> ("Modbus Master out"=w358:refnum<class "Modbus Master.lvclass">)
                n172 = call "inst.demux1.10(x6).vi"("demux1_10(x6)_encode"=T27."demux1_10_channel8", "Modbus Master in"=w358) -> ("error out"=w356:errorcluster)  [unwired: 8 in, 1 out]
              }
              frame condition #1 {
              }
            }
            n173 = Merge Errors(w354, w349) -> (w350:errorcluster)
          }
          frame "demux1-10_chan9" {
            n174 = Variant To Data(error in=w366, type=T20 {"Boolean"=FALSE} ("demux1-10_chan9 Argument"), Variant=w364) -> (error out=w365:errorcluster)  [unwired: 1 out]
            n175 = disable-structure shown="Default" {
              disable-tunnel: w362 -> [w370 _]
              disable-tunnel: [w367 _] -> w360
              frame condition #0 (active) {
                n176 = Unbundle By Name(w370) -> ("Modbus Master out"=w369:refnum<class "Modbus Master.lvclass">)
                n177 = call "inst.demux1.10(x6).vi"("demux1_10(x6)_encode"=T27."demux1_10_channel9", "Modbus Master in"=w369) -> ("error out"=w367:errorcluster)  [unwired: 8 in, 1 out]
              }
              frame condition #1 {
              }
            }
            n178 = Merge Errors(w365, w360) -> (w361:errorcluster)
          }
          frame "demux1-10_chan10" {
            n179 = Variant To Data(error in=w377, type=T21 {"Boolean"=FALSE} ("demux1-10_chan10 Argument"), Variant=w375) -> (error out=w376:errorcluster)  [unwired: 1 out]
            n180 = disable-structure shown="Default" {
              disable-tunnel: w373 -> [w381 _]
              disable-tunnel: [w378 _] -> w371
              frame condition #0 (active) {
                n181 = Unbundle By Name(w381) -> ("Modbus Master out"=w380:refnum<class "Modbus Master.lvclass">)
                n182 = call "inst.demux1.10(x6).vi"("demux1_10(x6)_encode"=T27."demux1_10_channel10", "Modbus Master in"=w380) -> ("error out"=w378:errorcluster)  [unwired: 8 in, 1 out]
              }
              frame condition #1 {
              }
            }
            n183 = Merge Errors(w376, w371) -> (w372:errorcluster)
          }
          frame "MB01_eMICs" {
            # "MB01 TurnON/OFF eMICs ( connect AC220V)"
            n184 = Variant To Data(error in=w389, type=T7 {"Array"=[FALSE, FALSE, FALSE, FALSE, FALSE, FALSE]} ("MB01_eMICs Argument"), Variant=w388) -> (data=w386:T7, error out=w383:errorcluster)
            n185 = disable-structure shown="NO_HARDWARE==TRUE" {
              disable-tunnel: w386 -> [w394 _]
              disable-tunnel: w385 -> [w393 _]
              disable-tunnel: [w390 _] -> w384
              frame condition #0 (active) {
                n186 = Unbundle By Name(w393) -> ("Modbus Master out"=w392:refnum<class "Modbus Master.lvclass">)
                n187 = Unbundle By Name(w394) -> ("Array"=w391:bool[])
                n188 = call "inst.MB Relay01(eMICs).vi"("MB relay01"=w391, "Modbus Master in"=w392) -> ("error out"=w390:errorcluster)  [unwired: 8 in, 1 out]
              }
              frame condition #1 {
              }
            }
            n189 = Merge Errors(w383, w384) -> (w382:errorcluster)
          }
          frame "SC enable OFF" {
            # "Turn +5V  OFF"
            n190 = Variant To Data(error in=w401, type=T11 {"Boolean"=FALSE} ("SC enable OFF Argument"), Variant=w399) -> (error out=w400:errorcluster)  [unwired: 1 out]
            n191 = disable-structure shown="Default" {
              disable-tunnel: w397 -> [w405 _]
              disable-tunnel: [w402 _] -> w395
              frame condition #0 (active) {
                n192 = Unbundle By Name(w405) -> ("Modbus Master out"=w404:refnum<class "Modbus Master.lvclass">)
                n193 = call "inst.SC enable.vi"("5V enable"=FALSE, "Modbus Master in"=w404) -> ("error out"=w402:errorcluster)  [unwired: 8 in, 1 out]
              }
              frame condition #1 {
              }
            }
            n194 = Merge Errors(w400, w395) -> (w396:errorcluster)
          }
          frame "JIG Reset" {
            # "Send Jig reset command to  release Fixture"
            n195 = disable-structure shown="Default" {
              disable-tunnel: w409 -> [w421 _]
              disable-tunnel: [w415 _] -> w406
              frame condition #0 (active) {
                n196 = Unbundle By Name(w421) -> ("Modbus Master out"=w420:refnum<class "Modbus Master.lvclass">)
                n197 = call "inst.JIG_RESET.vi"("JIG reset"=TRUE, "Modbus Master in"=w420) -> ("error out"=w418:errorcluster, "Modbus Master out"=w416:refnum<class "Modbus Master.lvclass">)  [unwired: 8 in]
                n198 = flat-sequence {
                  tunnel: [w423] -> w419
                  tunnel: w418 -> [w423]
                  tunnel: [w422] -> w417
                  tunnel: w416 -> [w422]
                  frame #0 {
                    n199 = Wait (ms)(milliseconds to wait=u32 300) -> ()  [unwired: 1 out]
                  }
                }
                n200 = call "inst.JIG_RESET.vi"("error in (no error)"=w419, "JIG reset"=FALSE, "Modbus Master in"=w417) -> ("error out"=w415:errorcluster)  [unwired: 7 in, 1 out]
              }
              frame condition #1 {
              }
            }
            n201 = Variant To Data(error in=w412, type=T9 {"Boolean"=FALSE} ("JIG Reset Argument"), Variant=w411) -> (error out=w408:errorcluster)  [unwired: 1 out]
            n202 = Merge Errors(w408, w406) -> (w407:errorcluster)
          }
          frame "Read JIG trigger" {
            # "Read JIG trigger value: pitton go down with generate triger signal, (return TRUE)"
            n203 = disable-structure shown="Default" {
              disable-tunnel: w427 -> [w441 _]
              disable-tunnel: [w439 _] -> w426
              disable-tunnel: [w438 w442] -> w425
              frame condition #0 (active) {
                n204 = Unbundle By Name(w441) -> ("Modbus Master out"=w440:refnum<class "Modbus Master.lvclass">)
                n205 = call "inst.JIG_TRIGGER.vi"("Modbus master in"=w440) -> ("error out"=w439:errorcluster, "JIG_TRIGGER"=w438:bool)  [unwired: 7 in, 2 out]
              }
              frame condition #1 {
                n206 = local read "trigger value"() -> (w442:bool)
              }
            }
            n207 = Variant To Data(error in=w437, type=T10 {"Wait Notifier"=refnum, "wait for reply"=FALSE} ("Read JIG trigger Argument"), Variant=w435) -> (data=w433:T10, error out=w436:errorcluster)
            n208 = Unbundle By Name(w433) -> ("Wait Notifier"=w432:refnum<notifier>, "wait for reply"=w431:bool)
            n209 = Bundle By Name(cluster=T28 {"Trigger?"=FALSE, "Read JIG trigger_error"={"status"=FALSE, "code"=0, "source"=""}} ("Read JIG trigger (Reply Payload)"), "Trigger?"=w425) -> (w430:T28)
            n210 = Merge Errors(w436, w426) -> (w428:errorcluster)
            n211 = case shown="True" w431 {
              tunnel: w432 -> [_ w444]
              tunnel: w430 -> [_ w443]
              frame False {
              }
              frame True {
                n212 = Send Notification(notification=w443, notifier=w444) -> ()  [unwired: 1 in, 2 out]
              }
            }
          }
          frame "SC enable ON" {
            n213 = Variant To Data(error in=w451, type=T22 {"Boolean"=FALSE} ("SC enable ON Argument"), Variant=w449) -> (error out=w450:errorcluster)  [unwired: 1 out]
            n214 = disable-structure shown="Default" {
              disable-tunnel: w447 -> [w455 _]
              disable-tunnel: [w453 _] -> w445
              frame condition #0 (active) {
                n215 = Unbundle By Name(w455) -> ("Modbus Master out"=w454:refnum<class "Modbus Master.lvclass">)
                n216 = call "inst.SC enable.vi"("5V enable"=TRUE, "Modbus Master in"=w454) -> ("error out"=w453:errorcluster)  [unwired: 8 in, 1 out]
              }
              frame condition #1 {
              }
            }
            n217 = Merge Errors(w450, w445) -> (w446:errorcluster)
          }
          frame "SET trigger value" {
            # "Set trigger value in Simulated mode"
            n218 = Variant To Data(error in=w462, type=T23 {"Boolean"=FALSE} ("SET trigger value Argument"), Variant=w459) -> (data=w457:T23, error out=w460:errorcluster)
            n219 = Unbundle By Name(w457) -> ("Boolean"=→"trigger value":bool)
          }
          frame "---Copy This Frame---" {
            # "Duplicate this frame when creating new messages.  Change this comment in the duplicated frame to describe this message."
            n220 = Merge Errors(w465) -> (w464:errorcluster)
          }
          frame "---Exit and Error Handling---" {
            # "Separator - The following cases handle errors and exit messages."
          }
          frame "Simulate MHL Error" {
            # "#DQMH_HowTo The 'Simulate MHL Error' button  illustrates how the MHL handles errors. This event is instructional in nature and can be removed."
            # "Simulate an error occurring at the MHL"
            n221 = call "Module Name--constant.vi"() -> ("Module Name"=w468:string)  [unwired: 11 in]
            n222 = xnode "Error Ring"("parameter 0"=w468) -> ("error out"=w470:errorcluster)
            n223 = Merge Errors(w472, w470) -> (w471:errorcluster)
          }
          frame "Error" {
            # "#CodeRecommended - If you ever change the name of this \"Error\" message, you'll need to update the name in the Check Loop Error.vi as well."
            # "#CodeRecommended - If the module is running in standalone mode (External Launch = FALSE), this code will pop up an error dialog and call the 'Exit' message if an error occurs. Add more fine-grained error handling here."
            # "Error - Check the error message data and respond accordingly. This message is sent by the \"Error Handler\" VIs at the end of each loop in this application."
            n224 = property class="Module Admin"(reference=w481) -> ("Accessors:External Launch"=w480:bool)  [unwired: 1 in, 2 out]
            n225 = Variant To Data(error in=w489, type=errorcluster {"status"=FALSE, "code"=0, "source"=""} ("error constant"), Variant=w483) -> (data=w490:errorcluster, error out=w487:errorcluster)
            n226 = call "Error Reported.vi"("Error"=w490) -> ()  [unwired: 10 in, 1 out]
            n227 = case shown="True" w480 {
              tunnel: [w495 _] -> w486
              tunnel: w482 -> [w493 _]
              tunnel: w490 -> [w494 _]
              frame False {
                # "If the module is running standalone, then pop up an error dialog and call the \"Exit\" message."
                n228 = call <vilib>:"Simple Error Handler.vi"("error in (no error)"=w494) -> ()  [unwired: 4 in, 5 out]
                n229 = call-poly <vilib>:"Delacor_lib_QMH_Enqueue Message (poly).vi"("Priority Message? (F)"=TRUE, "Message"="Exit", "Message Queue in"=w493) -> ("error out"=w495:errorcluster)  [unwired: 7 in, 1 out]
              }
              frame True {
                # "If the module was launched externally, calling the Error Reported broadcast VI is the only action performed by the \"Error\" message. The module's caller can then process the error appropriately."
              }
            }
            n230 = Merge Errors(w487, w486) -> (w485:errorcluster)
            n231 = local write "error out"(w485) -> ()
          }
          frame "Exit" {
            w502 = 91  # 91: not all Exit messages will have an argument
            w504 = TRUE  # Stop the VI
            # "Release the message queue reference"
            # "Exit - Exit the application."
            n232 = Variant To Data(error in=w511, type=T4 {"Origin"="", "Exit via Stop Module Req?"=FALSE, "Wait for Module to stop?"=FALSE} ("Stop Argument"), Variant=w503) -> (data=w500:T4, error out=w507:errorcluster)
            n233 = disable-structure shown="NO_HARDWARE==TRUE" {
              disable-tunnel: w497 -> [w517 _]
              disable-tunnel: [w516 _] -> w496
              frame condition #0 (active) {
                n234 = Unbundle By Name(w517) -> ("Modbus Master out"=w515:refnum<class "Modbus Master.lvclass">)
                n235 = call "FGV_HoldingRegs.vi"("FGV_enum"=FGV_enum."All OFF", "Modbus master in"=w515) -> ("error out"=w513:errorcluster, "Modbus master out"=w512:refnum<class "Modbus Master.lvclass">)  [unwired: 7 in, 1 out]
                n236 = call "inst.Close (SubVI).vi"("error in (no error)"=w513, "Modbus Master in"=w512) -> ("error out"=w516:errorcluster)  [unwired: 9 in]
              }
              frame condition #1 {
              }
            }
            n237 = call <vilib>:"Clear Errors.vi"("error in (no error)"=w507, "specific error code to clear (0: all)"=w502) -> ("error out"=w510:errorcluster)  [unwired: 4 in, 1 out]
            n238 = control-ref of="This VI"() -> (w499:refnum<vi>)
            n239 = call-dynamic "Delacor_lib_QMH_Release Message Queue.vi"("error in"=w510, "Message Queue"=w505) -> ("error out"=w509:errorcluster)  [unwired: 9 in]
            n240 = call "Handle Exit.vi"("Stop Argument"=w500, "Admin in"=w498, "VI reference"=w499) -> ("error out"=w506:errorcluster)  [unwired: 7 in, 1 out]
            n241 = Merge Errors(w509, w506, w496) -> (w508:errorcluster)
          }
          frame Default {
            # "'Default' case only runs if there is a message that isn't defined in any of the other cases.  Output a programming error."
            n242 = call "Module Name--constant.vi"() -> ("Module Name"=w518:string)  [unwired: 11 in]
            n243 = xnode "Error Ring"("parameter 0"=w519, "parameter 1"=w518) -> ("error out"=w523:errorcluster)
            n244 = Merge Errors(w521, w523) -> (w522:errorcluster)
          }
        }
        n245 = call-dynamic "Delacor_lib_QMH_Error Handler - Message Handling Loop.vi"("error in"=w208, "Message Queue in"=w198) -> ("dup error in"=w205:errorcluster)  [unwired: 8 in, 1 out]
      }
    }
    frame Error {
      # "Synchronize Caller Events.vi will inform Start Module.vi that the module has launched and will let the code calling Start Module.vi register for broadcasts and would permit the caller receive the broadcast that an error occurred at launch time."
      n246 = call-dynamic "Delacor_lib_QMH_Release Message Queue.vi"("error in"=w534, "Message Queue"=w532) -> ("error out"=w533:errorcluster)  [unwired: 9 in]
      n247 = call "Synchronize Caller Events.vi"("Singleton Module Admin in"=w535) -> ("error out"=w540:errorcluster)  [unwired: 9 in, 1 out]
      n248 = call "Module Name--constant.vi"() -> ("Module Name"=w538:string)  [unwired: 11 in]
      n249 = Format Into String(format string="An error occurred during initialization. %s is no longer running.", w538) -> (resulting string=w536:string)  [unwired: 2 in, 1 out]
      n250 = Merge Errors(w533, w540) -> (w541:errorcluster)
      n251 = call "Error Reported.vi"("Additional Information"=w536, "Error"=w541) -> ()  [unwired: 9 in, 1 out]
    }
  }
  n252 = Merge Errors(w14, w17) -> (w13:errorcluster)
  n253 = call "Close Module.vi"("error in (no error)"=w13, "Module Admin in"=w8) -> ("error out"=w15:errorcluster, "External Launch"=w1:bool, "Module Admin out"=w2:refnum<class "Delacor_lib_QMH_Module Admin.lvclass">)  [unwired: 7 in]
  n254 = Unregister For Events(event registration refnum=w7, error in=w15) -> (error out=w12:errorcluster)
  "error out" <- w12
  n255 = case "External Launch?" shown="True" w1 {
    tunnel: w12 -> [_ w542]
    frame False {
    }
    frame True {
      n256 = case shown="No Error" w542 {
        frame No Error {
          n257 = invoke class="VI" method="FP.Close"() -> ()  [unwired: 3 in, 3 out]
        }
        frame Error {
          n258 = invoke class="VI" method="FP.Open"("Activate"=TRUE ("Activate?")) -> ()  [unwired: 4 in, 5 out]
        }
      }
    }
  }
  n259 = local write "Module Admin"(w2) -> ()
